vi "MCP2221_Sample.vi"() -> ()   [LabVIEW 2025]
panel:
  out "gpio direction":bool[](array[boolean])
  in  "gpio direction":bool[](array[boolean])=[FALSE, FALSE, FALSE, FALSE]
  out "gpio value":bool[](array[boolean])
  in  "gpio value":bool[](array[boolean])=[FALSE, FALSE, FALSE, FALSE]
  out "error out":errorcluster
  # "SET"
  # "GET"
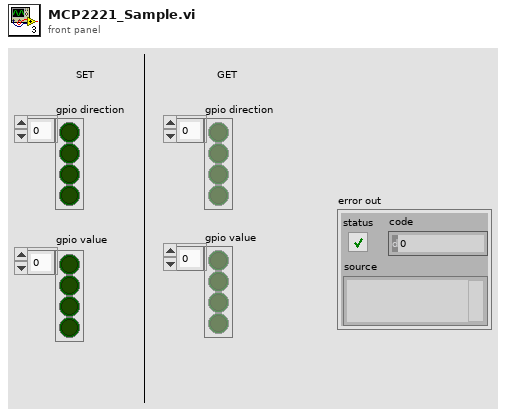
[diagram p1: front panel]
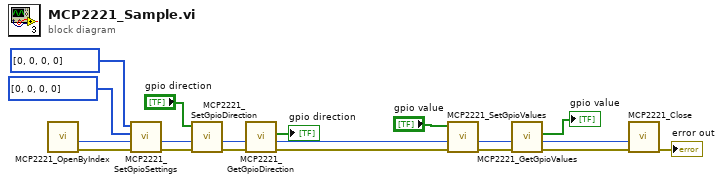
[diagram p0: block diagram]
diagram:
  n1 = call "MCP2221_OpenByIndex.vi"() -> ("error out"=w1:errorcluster, "handle out"=w2:i32)  [unwired: 10 in]
  n2 = call "MCP2221_SetGpioSettings.vi"("error in"=w1, "handle in"=w2, "outputValues"=u8[] [0, 0, 0, 0], "pinDirections"=u8[] [0, 0, 0, 0]) -> ("error out"=w12:errorcluster, "handle out"=w19:i32)  [unwired: 5 in, 1 out]
  n3 = call "MCP2221_SetGpioDirection.vi"("error in"=w12, "handle in"=w19, "direction"="gpio direction") -> ("error out"=w11:errorcluster, "handle out"=w18:i32)  [unwired: 6 in, 1 out]
  n4 = call "MCP2221_GetGpioDirection.vi"("error in"=w11, "handle in"=w18) -> ("error out"=w10:errorcluster, "handle out"=w17:i32, "direction"=→"gpio direction":bool[])  [unwired: 6 in, 1 out]
  n5 = call "MCP2221_SetGpioValues.vi"("error in"=w10, "handle in"=w17, "gpio"="gpio value") -> ("error out"=w9:errorcluster, "handle out"=w16:i32)  [unwired: 6 in, 1 out]
  n6 = call "MCP2221_GetGpioValues.vi"("error in"=w9, "handle in"=w16) -> ("error out"=w7:errorcluster, "handle out"=w15:i32, "gpio"=→"gpio value":bool[])  [unwired: 6 in, 1 out]
  n7 = call "MCP2221_Close.vi"("error in"=w7, "handle in"=w15) -> ("error out"=→"error out":errorcluster)  [unwired: 7 in, 2 out]
